vi "CreateHardwareDataStructures.vi"(8 "Error In":errorcluster) -> (0 "Error Out":errorcluster, 3 "Hardware Data Structures":T1)   [LabVIEW 2012]
uses:
  HardwareDataStructures.ctl
  PXI6229Data.ctl
  CurrentMeterData.ctl
  HardwareLogData.ctl
  HardwareDisplayData.ctl
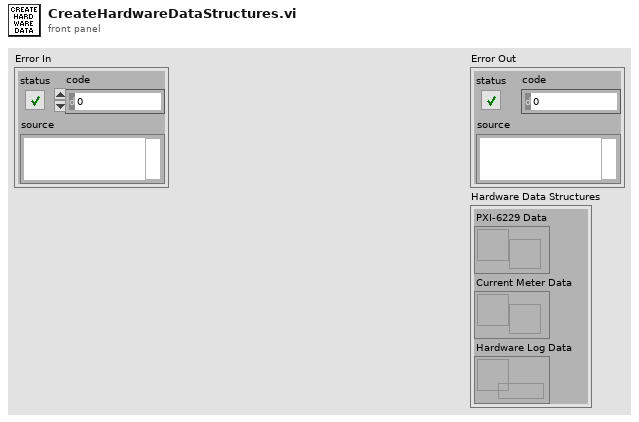
[diagram p1: front panel]
types:
  T1 = typedef "HardwareDataStructures.ctl" = cluster{"PXI-6229 Data":refnum<notifier>, "Current Meter Data":refnum<notifier>, "Hardware Log Data":refnum<queue>}
  T2 = typedef "CurrentMeterData.ctl" = dbl[]
  T3 = typedef "HardwareLogData.ctl" = cluster{"Time Stamp":timestamp, "Data":T4}
  T4 = typedef "HardwareDisplayData.ctl" = cluster{"Temperatures (C)":dbl[], "Terminal Voltage (MeV)":dbl, "Currents (A)":dbl[]}
  T5 = typedef "PXI6229Data.ctl" = cluster{"Temperatures":dbl[][], "Terminal Voltage":dbl[][], "BPM":dbl[][]}
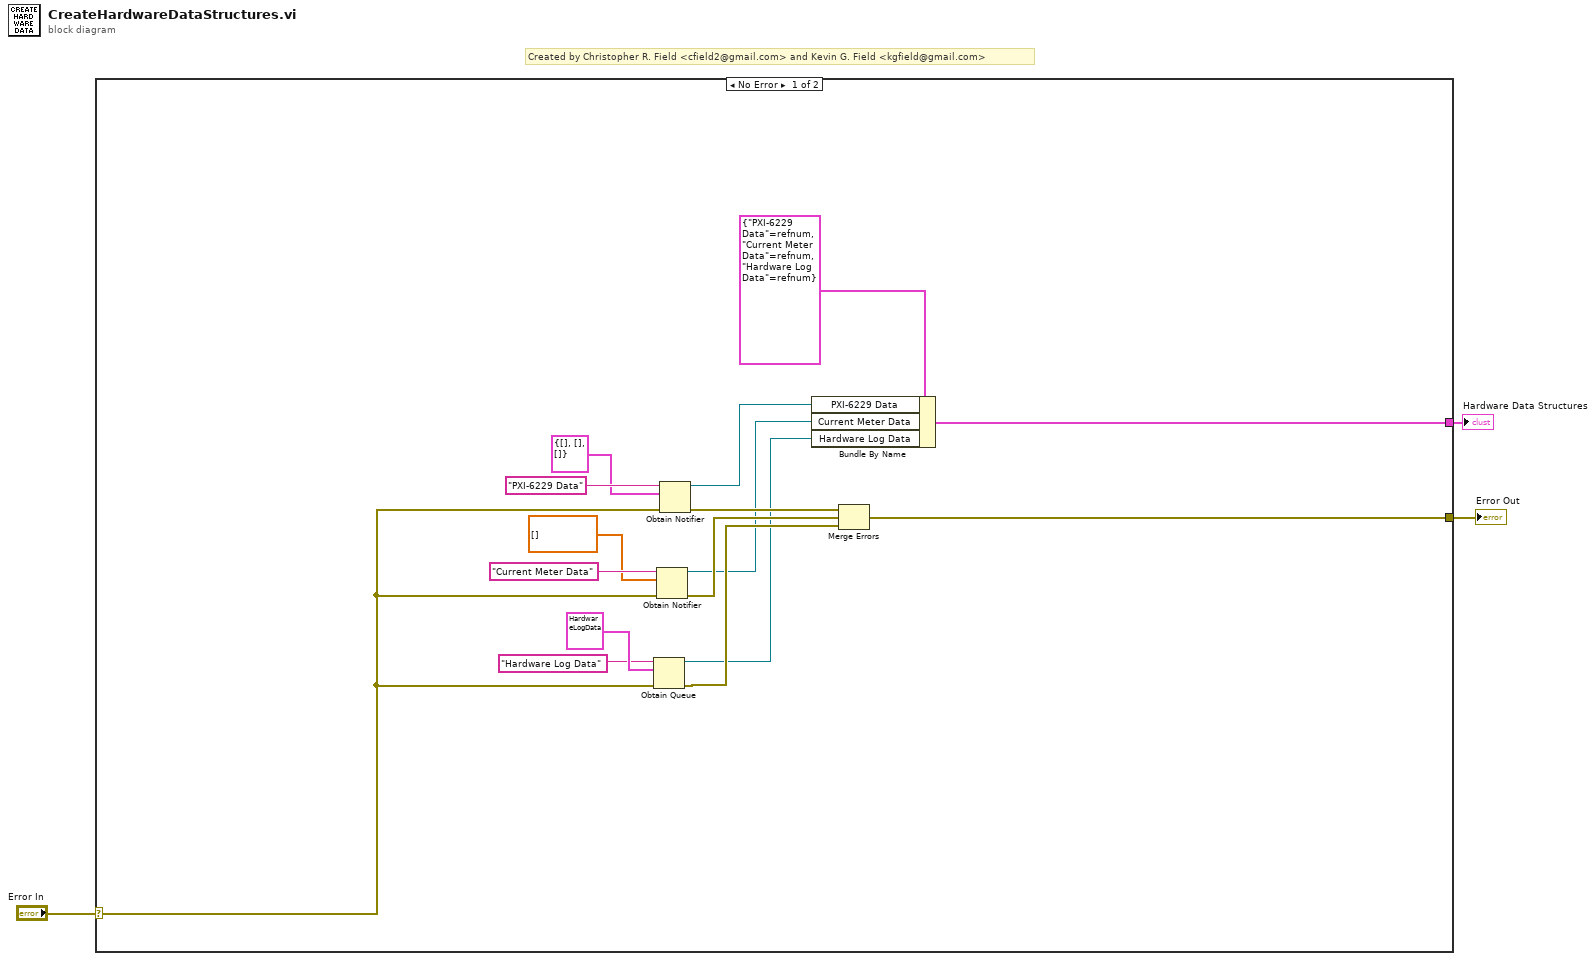
[diagram p0: block diagram]
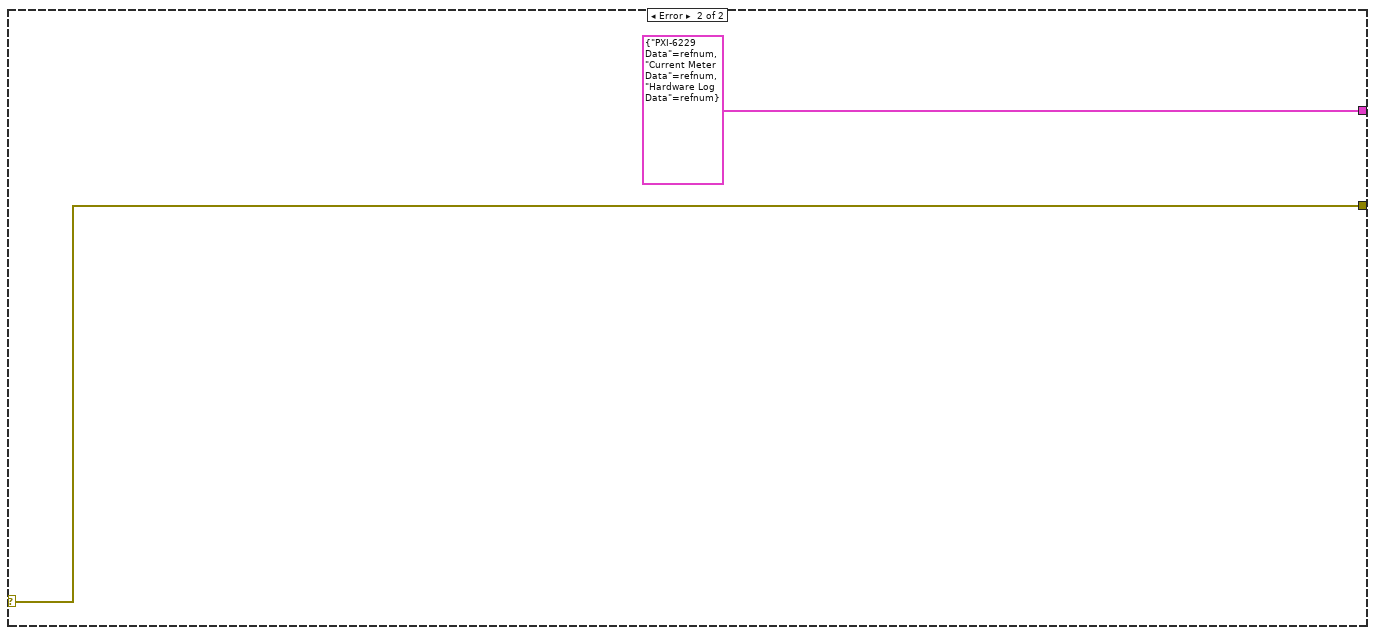
[diagram p2: hidden frame]
diagram:
  # "Created by Christopher R. Field <cfield2@gmail.com> and Kevin G. Field <kgfield@gmail.com>"
  n1 = case shown="No Error" "Error In" {
    selector: "Error In" -> [w14 w21]
    tunnel: [w10 w21] -> w2
    tunnel: [w6 T1 {"PXI-6229 Data"=refnum, "Current Meter Data"=refnum, "Hardware Log Data"=refnum} ("Hardware Data Structures")] -> w1
    frame No Error {
      n2 = Obtain Queue(name (unnamed)="Hardware Log Data", element data type=T3 {"Time Stamp"=timestamp(0 s since 1904-01-01), "Data"={"Temperatures (C)"=[], "Terminal Voltage (MeV)"=0.0, "Currents (A)"=[]}} ("Hardware Log Data Queue Element"), error in (no error)=w14) -> (queue out=w7:refnum<queue>, error out=w11:errorcluster)  [unwired: 2 in, 1 out]
      n3 = Obtain Notifier(name (unnamed)="Current Meter Data", notification data type=T2 [] ("Current Meter Data"), error in (no error)=w14) -> (notifier out=w4:refnum<notifier>, error out=w12:errorcluster)  [unwired: 1 in, 1 out]
      n4 = Obtain Notifier(name (unnamed)="PXI-6229 Data", notification data type=T5 {"Temperatures"=[], "Terminal Voltage"=[], "BPM"=[]} ("DAQ Data Queue Element"), error in (no error)=w14) -> (notifier out=w8:refnum<notifier>, error out=w13:errorcluster)  [unwired: 1 in, 1 out]
      n5 = Bundle By Name(cluster=T1 {"PXI-6229 Data"=refnum, "Current Meter Data"=refnum, "Hardware Log Data"=refnum} ("Hardware Data Structures"), "PXI-6229 Data"=w8, "Current Meter Data"=w4, "Hardware Log Data"=w7) -> (w6:T1)
      n6 = Merge Errors(w13, w12, w11) -> (w10:errorcluster)
    }
    frame Error {
    }
  }
  "Error Out" <- w2
  "Hardware Data Structures" <- w1
